vi "Normal Mode.vi"(8 "error in (no error)":errorcluster) -> (0 "error out":errorcluster)   [LabVIEW 2023, in "Internal Communication.lvlib"]
doc: "Send normal mode state to all queues"
uses:
  Internal Communication.lvlib
  Controls/State FGV.ctl
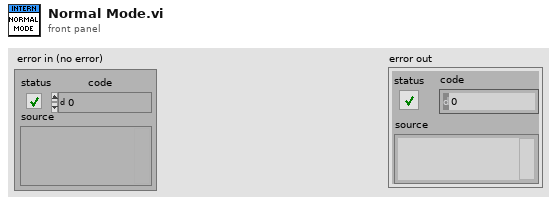
[diagram p1: front panel]
types:
  T1 = typedef "Internal Communication.lvlib/State FGV.ctl" = enum16{"Create Queues", "Get Queues", "Destroy Queues"}
  T2 = typedef "Internal Communication.lvlib/Queues Control.ctl" = cluster{"Heart":refnum<queue>, "FPGA":refnum<queue>, "Encoder":refnum<queue>, "Decoder":refnum<queue>, "Error":refnum<queue>, "UI":refnum<queue>}
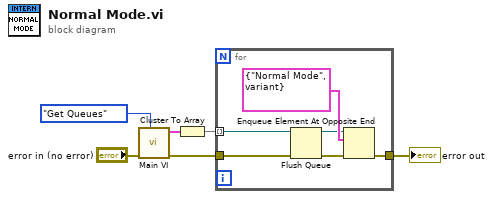
[diagram p0: block diagram]
diagram:
  n1 = call "Main VI.vi"("Enum"=State_FGV."Get Queues", "error in (no error)"="error in (no error)") -> ("error out"=w2:errorcluster, "Queues"=w5:T2)  [unwired: 8 in]
  n2 = Cluster To Array(cluster=w5) -> (array=w4:refnum<queue>[])
  n3 = for {
    tunnel: w4 -> [w10] mode=indexing
    tunnel: w2 -> [w8]
    tunnel: [w11] -> w1
    n4 = Flush Queue(queue=w10, error in (no error)=w8) -> (queue out=w9:refnum<queue>, error out=w7:errorcluster)  [unwired: 1 out]
    n5 = Enqueue Element At Opposite End(queue=w9, element=cluster{string, variant} {"Normal Mode", variant}, error in (no error)=w7) -> (error out=w11:errorcluster)  [unwired: 1 in, 2 out]
  }
  "error out" <- w1
